vi "Time_string.vi"(11 "h in":timestamp) -> (2 "heure sql":string, 3 "date":string)   [LabVIEW 2020]
panel:
  # "2022-08-23 16:19:54"
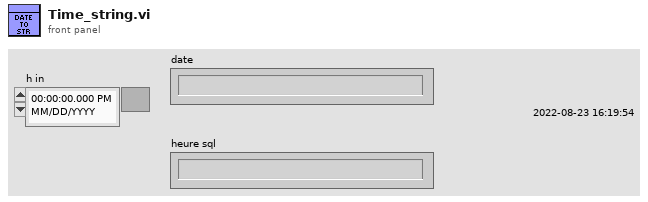
[diagram p1: front panel]
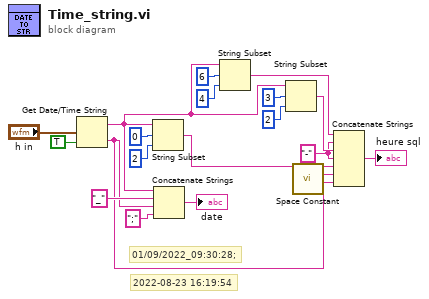
[diagram p0: block diagram]
diagram:
  w1 = "-"
  # "01/09/2022_09:30:28;"
  # "2022-08-23 16:19:54"
  n1 = Get Date/Time String(seconds (now)="h in", want seconds? (F)=TRUE ("secondes ? (F)")) -> (date string=w16:string, time string=w4:string)  [unwired: 1 in]
  n2 = String Subset(string=w16, offset (0)=0, length (rest)=2 ("longueur (reste)")) -> (substring=w7:string)
  n3 = Concatenate Strings(w16, "_" ("chaîne"), w4, ";" ("chaîne")) -> (→"date":string)
  n4 = String Subset(string=w16, offset (0)=6, length (rest)=4 ("longueur (reste)")) -> (substring=w9:string)
  n5 = String Subset(string=w16, offset (0)=3, length (rest)=2 ("longueur (reste)")) -> (substring=w8:string)
  n6 = call <vilib>:"Space Constant.vi"() -> ("String"=w5:string)
  n7 = Concatenate Strings(w9, w1, w8, w1, w7, w5, w4) -> (→"heure sql":string)
